vi "mx28mon.vi"() -> ()   [LabVIEW 2018]
uses:
  <vilib>/Platform/TimedLoop/XDataNode/timing_clust.ctl
  <vilib>/Platform/TimedLoop/XDataNode/nitl_modes.ctl
  <vilib>/Platform/TimedLoop/XDataNode/wakeup.ctl
  <vilib>/Platform/TimedLoop/XDataNode/XDataNode.xnode
  <vilib>/Platform/TimedLoop/XDataNode/XDNodeRunTimeDep.lvlib
panel:
  out "tick":u32
  out "停止":bool
  out "err":u32
  out "出力クラスタ":T1
  out "波形チャート":T1(graph)
  in  "Baudrate":u32=2000000
  in  "COM":refnum<visa-resource-name>="COM5" caption="COMポート"
  in  "STOP":bool
  in  "GOAL POSITION":i16(knob) scale=20.0..4075.0
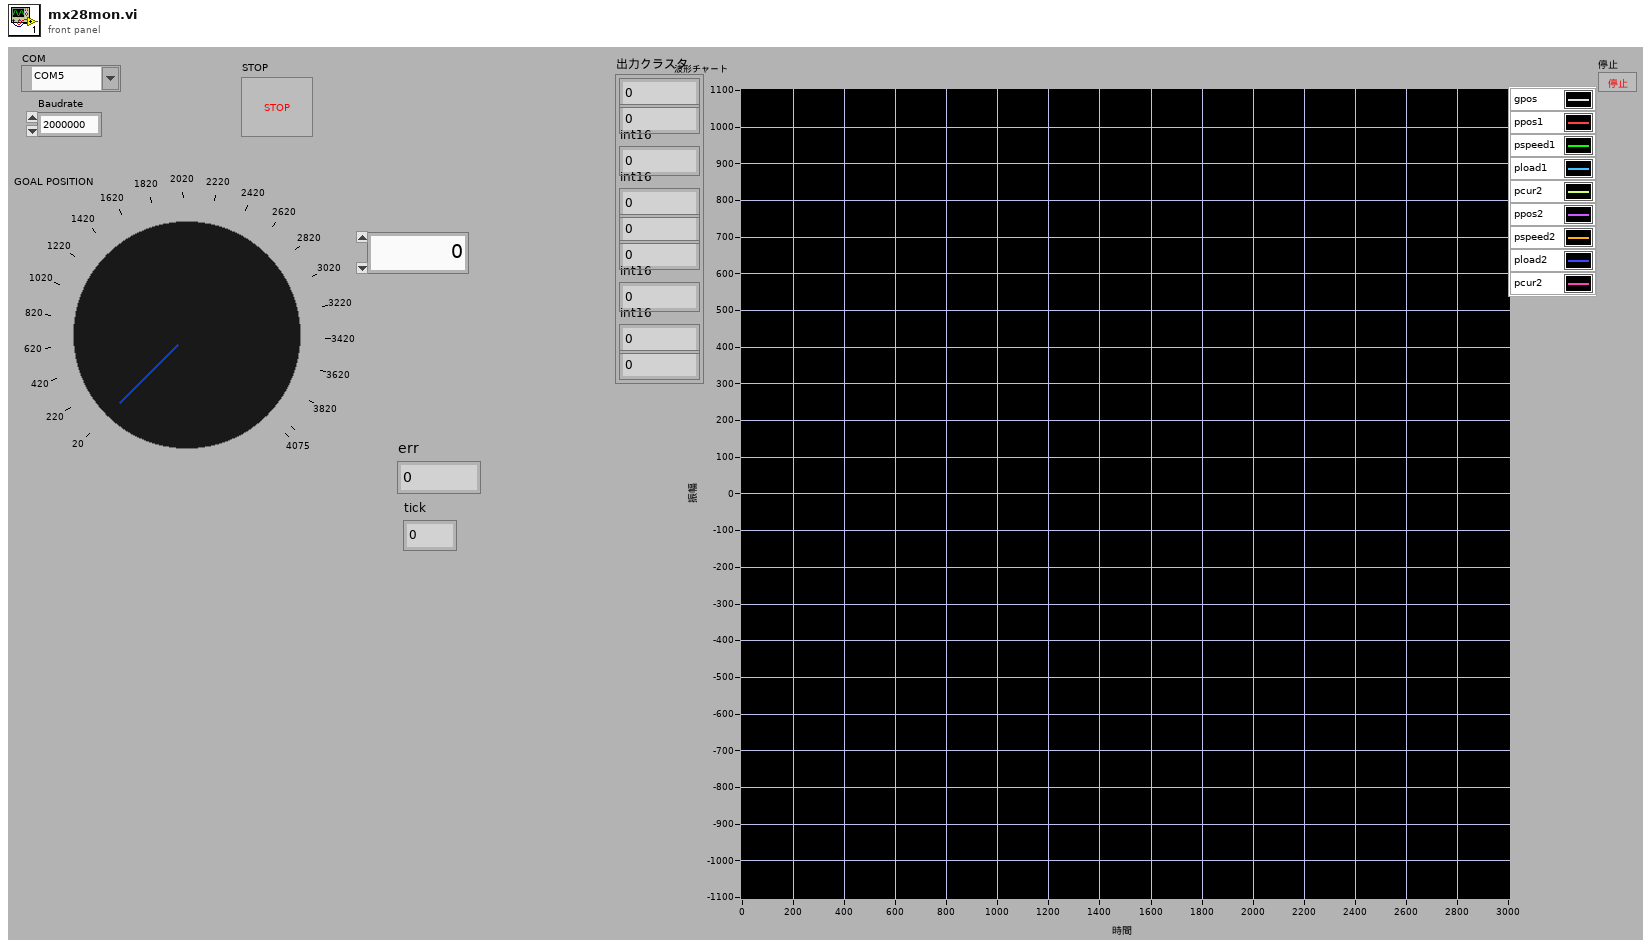
[diagram p1: front panel]
types:
  T1 = cluster{dbl, dbl, "int16":i16, "int16":i16, dbl, dbl, "int16":i16, "int16":i16, dbl}
  T2 = typedef "XDNodeRunTimeDep.lvlib/timing_clust.ctl" = cluster{"Expected End [f-1]":u64, "Actual End [f-1]":u64, "Finished Late? [f-1]":bool, "Expected End [i-1]":u64, "Actual End [i-1]":u64, "Finished Late? [i-1]":bool, "Expected Start [i]":u64, "Actual Start [i]":u64, "Expected Start [f]":u64, "Actual Start [f]":u64, "Source Name":string, "Structure Name":string, "Period":i64, "Deadline":i64, "Offset":i64, "Start":i64, "Priority":i32, "Timeout":i32, "Mode":T3, "Wakeup Reason":T4, "Error":errorcluster, "Source Type":string, "Secondary Source Type":string, "Global End Time":u64, "Global Start Time":u64, "Frame Duration":u64, "Iteration Duration":u64, "Assigned CPU":i32, "I/O Scan Engine Mode":u32}
  T3 = typedef "XDNodeRunTimeDep.lvlib/nitl_modes.ctl" = enum32{"No Change", "Process missed periods, maintain original phase", "Discard missed periods, maintain original phase", "Process missed periods, ignore original phase", "Discard missed periods, ignore original phase"}
  T4 = typedef "XDNodeRunTimeDep.lvlib/wakeup.ctl" = enum32{"Normal", "Aborted", "Asynchronous wakeup", "Timing source error", "Timed loop error", "Timeout"}
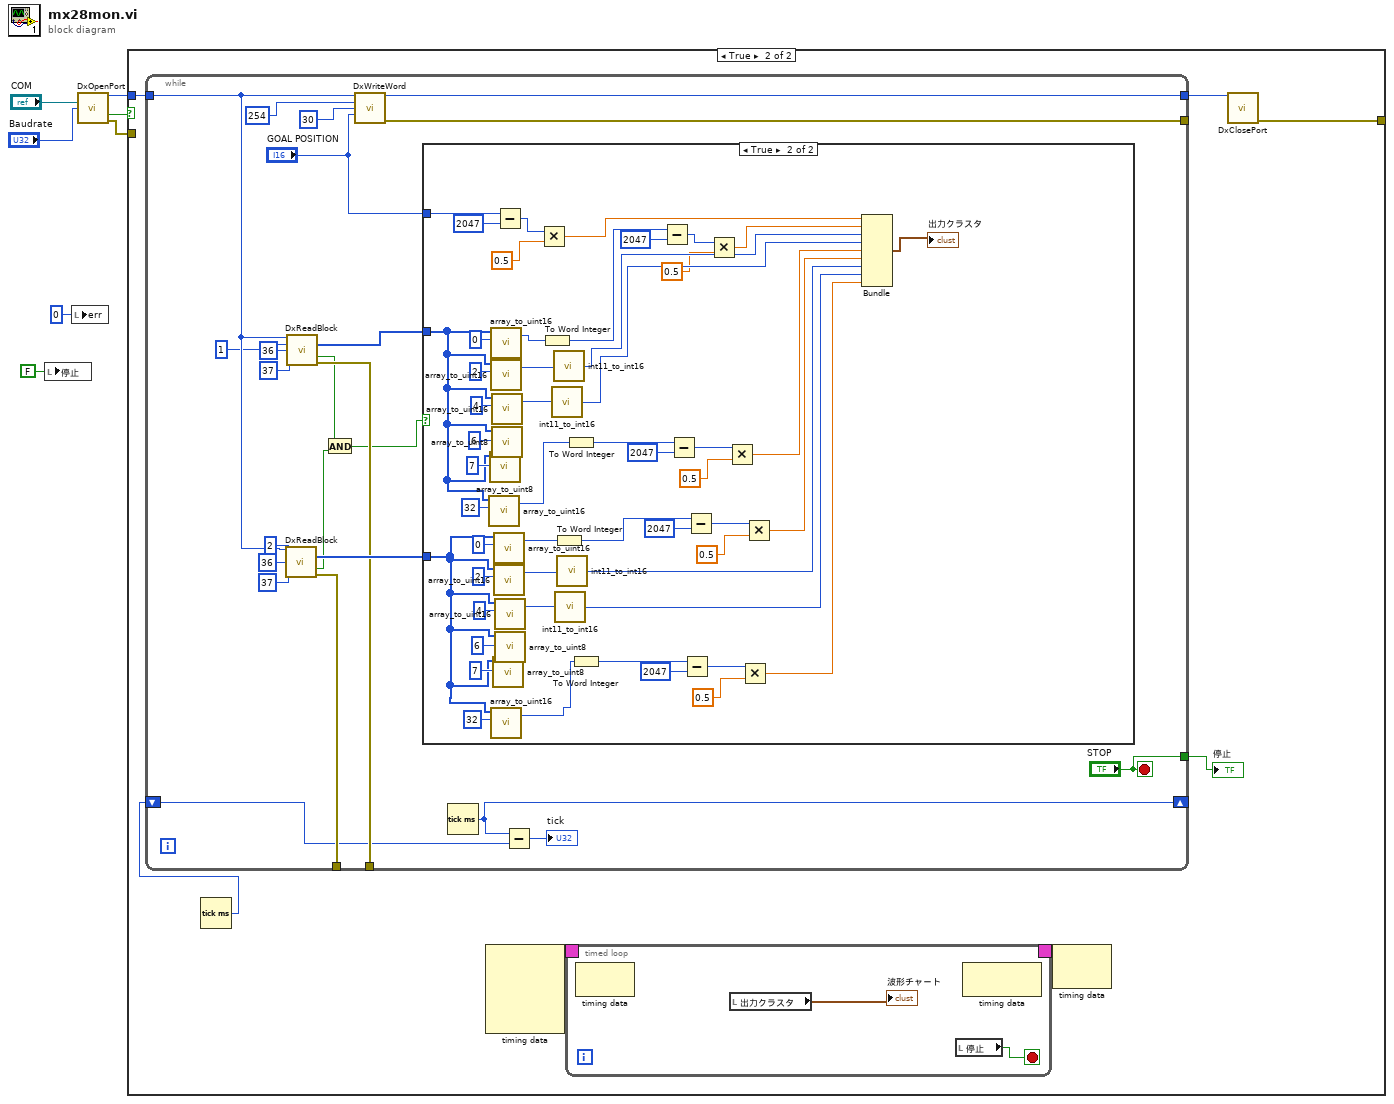
[diagram p0: block diagram]
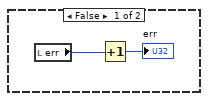
[diagram p3: hidden frame]
diagram:
  n1 = local write "停止"(FALSE ("停止")) -> ()
  n2 = local write "err"(u32 0 ("err")) -> ()
  n3 = call "DxOpenPort.vi"("port"="COM", "baudrate"="Baudrate") -> ("dvid"=w5:u32, "成功"=w4:bool, "エラー出力"=w3:errorcluster)  [unwired: 11 in]
  n4 = case shown="TRUE" w4 {
    tunnel: w5 -> [_ w14]
    tunnel: w3 -> [_ _]
    tunnel: [_ w12] -> _
    frame False {
    }
    frame True {
      n5 = Tick Count (ms)() -> (millisecond timer value=w8:u32)
      n6 = while {
        tunnel: w14 -> [w34]
        tunnel: [w42] -> w13
        tunnel: [w41] -> _
        tunnel: [w29] -> _
        tunnel: [w28] -> _
        tunnel: ["STOP"] -> w9
        shift-right: [w22] -> _
        shift-left: w8 -> [w23]
        stop <- "STOP" stop-if-true
        n7 = call "DxReadBlock.vi"("dvid in"=w34, "id"=u8 2, "address"=u16 36, "size"=u32 37) -> ("data out"=w30:u8[], "成功"=w26:bool, "エラー出力"=w28:errorcluster)  [unwired: 8 in, 1 out]
        n8 = call "DxReadBlock.vi"("dvid in"=w34, "id"=u8 1, "address"=u16 36, "size"=u32 37) -> ("data out"=w38:u8[], "成功"=w27:bool, "エラー出力"=w29:errorcluster)  [unwired: 8 in, 1 out]
        n9 = And(x=w27, y=w26) -> (x .and. y?=w25:bool)
        n10 = call "DxWriteWord.vi"("dvid in"=w34, "id"=u8 254, "address"=u16 30, "data in"="GOAL POSITION") -> ("dvid out"=w42:u32, "エラー出力"=w41:errorcluster)  [unwired: 9 in, 1 out]
        n11 = case shown="TRUE" w25 {
          tunnel: w38 -> [_ w60]
          tunnel: "GOAL POSITION" -> [_ w90]
          tunnel: w30 -> [_ w58]
          frame False {
            n12 = local read "err"() -> (w44:u32)
            n13 = Increment(x=w44) -> (x+1=→"err":u32)
          }
          frame True {
            n14 = call "array_to_uint16.vi"("OffsetAddr"=u16 32, "array"=w60) -> ("uint16"=w50:u16)  [unwired: 5 in]
            n15 = call "array_to_uint8.vi"("OffsetAddr"=u16 7, "array"=w60) -> ()  [unwired: 5 in, 1 out]
            n16 = call "array_to_uint16.vi"("OffsetAddr"=u16 0, "array"=w60) -> ("uint16"=w75:u16)  [unwired: 5 in]
            n17 = call "array_to_uint16.vi"("OffsetAddr"=u16 2, "array"=w60) -> ("uint16"=w93:u16)  [unwired: 5 in]
            n18 = call "array_to_uint16.vi"("OffsetAddr"=u16 32, "array"=w58) -> ("uint16"=w48:u16)  [unwired: 5 in]
            n19 = call "array_to_uint16.vi"("OffsetAddr"=u16 4, "array"=w60) -> ("uint16"=w92:u16)  [unwired: 5 in]
            n20 = call "array_to_uint8.vi"("OffsetAddr"=u16 6, "array"=w60) -> ()  [unwired: 5 in, 1 out]
            n21 = call "array_to_uint8.vi"("OffsetAddr"=u16 7, "array"=w58) -> ()  [unwired: 5 in, 1 out]
            n22 = call "array_to_uint16.vi"("OffsetAddr"=u16 0, "array"=w58) -> ("uint16"=w76:u16)  [unwired: 5 in]
            n23 = call "array_to_uint16.vi"("OffsetAddr"=u16 2, "array"=w58) -> ("uint16"=w87:u16)  [unwired: 5 in]
            n24 = Subtract(x=w90, y=i16 2047) -> (x-y=w70:i16)
            n25 = call "array_to_uint16.vi"("OffsetAddr"=u16 4, "array"=w58) -> ("uint16"=w88:u16)  [unwired: 5 in]
            n26 = call "array_to_uint8.vi"("OffsetAddr"=u16 6, "array"=w58) -> ()  [unwired: 5 in, 1 out]
            n27 = Multiply(x=w70, y=0.5) -> (x*y=w69:dbl)
            n28 = To Word Integer(number=w75) -> (16bit integer=w74:i16)
            n29 = call "int11_to_int16.vi"("int11"=w92) -> ("int16"=w71:i16)
            n30 = call "int11_to_int16.vi"("int11"=w93) -> ("int16"=w72:i16)
            n31 = To Word Integer(number=w76) -> (16bit integer=w73:i16)
            n32 = call "int11_to_int16.vi"("int11"=w88) -> ("int16"=w81:i16)
            n33 = call "int11_to_int16.vi"("int11"=w87) -> ("int16"=w82:i16)
            n34 = To Word Integer(number=w50) -> (16bit integer=w46:i16)
            n35 = To Word Integer(number=w48) -> (16bit integer=w47:i16)
            n36 = Subtract(x=w74, y=i16 2047) -> (x-y=w66:i16)
            n37 = Subtract(x=w46, y=i16 2047) -> (x-y=w57:i16)
            n38 = Subtract(x=w47, y=i16 2047) -> (x-y=w52:i16)
            n39 = Subtract(x=w73, y=i16 2047) -> (x-y=w63:i16)
            n40 = Multiply(x=w66, y=0.5) -> (x*y=w65:dbl)
            n41 = Multiply(x=w57, y=0.5) -> (x*y=w49:dbl)
            n42 = Multiply(x=w52, y=0.5) -> (x*y=w51:dbl)
            n43 = Multiply(x=w63, y=0.5) -> (x*y=w62:dbl)
            n44 = Bundle(w69, w65, "int16"=w72, "int16"=w71, w49, w62, "int16"=w82, "int16"=w81, w51) -> (→"出力クラスタ":T1)  [unwired: 1 in]
          }
        }
        n45 = Tick Count (ms)() -> (millisecond timer value=w22:u32)
        n46 = Subtract(x=w22, y=w23) -> (x-y=→"tick":u32)
      }
      "停止" <- w9
      n47 = node-c288() -> (w11:T2)  [unwired: 4 in]
      n48 = timed-loop {
        timing: w11 -> [_]
        timing-out: [_] -> w10
        stop <- w15 stop-if-true
        n49 = node-c288() -> ()  [unwired: 1 in, 1 out]
        n50 = local read "出力クラスタ"() -> (→"波形チャート":T1)
        n51 = local read "停止"() -> (w15:bool)
        n52 = node-c288() -> ()  [unwired: 1 in, 1 out]
      }
      n53 = node-c288(w10) -> ()  [unwired: 1 out]
      n54 = call "DxClosePort.vi"("dvid"=w13) -> ("エラー出力"=w12:errorcluster)  [unwired: 13 in, 1 out]
    }
  }
